vi "快捷键电阻单次采集.vi"(6 "数据显示1":string[][](table), 9 "Coords":T1, 10 "CtlRef":refnum<vi>, 11 "Keithley2705":refnum<visa-resource-name>) -> (0 "采集值+平均值":string[](array[string]), 2 "数据显示2":string[][](table), 4 "完成对话框":string)   [LabVIEW 2015]
uses:
  <vilib>/Utility/miscctls.llb/LVPoint32TypeDef.ctl
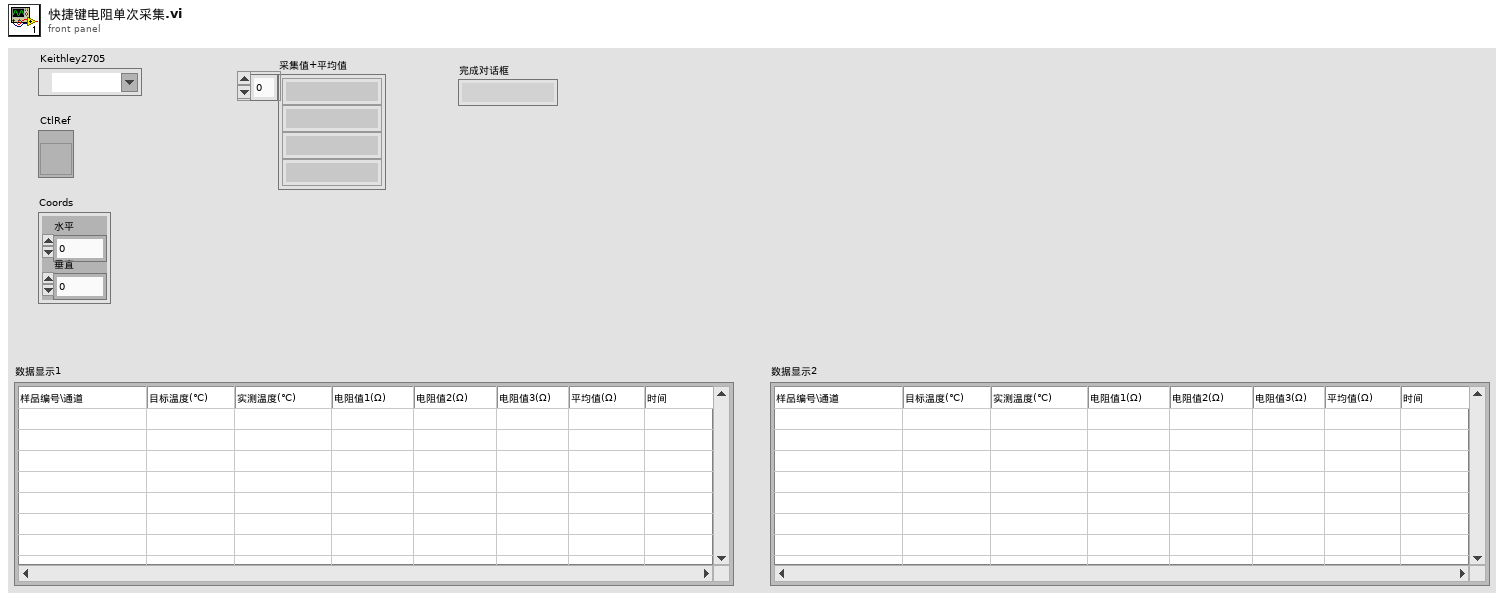
[diagram p1: front panel]
types:
  T1 = typedef "LVPoint32TypeDef.ctl" = cluster{"Horizontal":i32, "Vertical":i32}
  T2 = typedef "LVRowAndColumnTypeDef.ctl" = cluster{"Row":i32, "Column":i32}
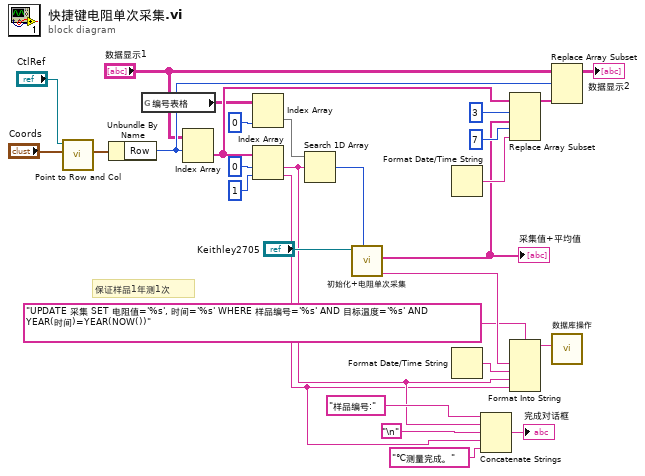
[diagram p0: block diagram]
diagram:
  # "保证样品1年测1次"
  n1 = call "Point to Row and Col.vi"("点"="Coords", "Table Ref In"="CtlRef") -> ("单元格位置"=w29:T2)  [unwired: 6 in, 3 out]
  n2 = Unbundle By Name(w29) -> ("Row"=w13:i32)
  n3 = global read "全局.vi" "编号表格"() -> (w10:string[][])
  n4 = Index Array(array="数据显示1", index (row)=w13) -> (element=w20:string[])  [unwired: 1 in]
  n5 = Index Array(array=w10, index (col)=0 ("禁用的索引 (列)")) -> (element=w12:string[])  [unwired: 1 in]
  n6 = Index Array(array=w20, index #1=0 ("索引"), index #2=1 ("索引")) -> (element #1=w5:string, element #2=w3:string)
  n7 = Search 1D Array(1D array=w12, element=w5) -> (index of element=w19:i32)  [unwired: 1 in]
  n8 = call "初始化+电阻单次采集.vi"("通道号"=w19, "VISA引用句柄输入"="Keithley2705") -> ("平均值"=w24:string, "采集值+平均值"=w15:string[])  [unwired: 8 in]
  "采集值+平均值" <- w15
  n9 = Format Date/Time String() -> (date/time string=w17:string)  [unwired: 3 in]
  n10 = Format Date/Time String() -> (date/time string=w26:string)  [unwired: 3 in]
  n11 = Concatenate Strings("样品编号:", w5, "\n", w3, "℃测量完成。") -> (→"完成对话框":string)
  n12 = Replace Array Subset(array=w20, new element #1=w15, index #1=3 ("索引"), new element #2=w17, index #2=7 ("索引")) -> (w18:string[])
  n13 = Format Into String(format string="UPDATE 采集 SET 电阻值='%s', 时间='%s' WHERE 样品编号='%s' AND 目标温度='%s' AND YEAR(时间)=YEAR(NOW())" ("SQL"), w24, w26, w5, w3) -> (resulting string=w22:string)  [unwired: 2 in, 1 out]
  n14 = Replace Array Subset(array="数据显示1", new element=w18, index (row)=w13) -> (→"数据显示2":string[][])  [unwired: 1 in]
  n15 = call "数据库操作.vi"("SQL query"=w22) -> ()  [unwired: 9 in, 2 out]
